vi "FA_Open.vi"(7 "LSCollections":T1, 8 "Error In":errorcluster, 10 "Special Types Array":T2[](array[typedef])) -> (0 "Error Out":errorcluster, 3 "FA_LS Ref":T3)   [LabVIEW 2014, in "FA_LocalStore.lvlib"]
doc: "Opens a reference to the XML files for each Special Type configuraiton. Implicitely opens reference to FA_eTag."
uses:
  FA_LocalStore.lvlib
  FA_LSRef.ctl
  <vilib>/Utility/config.llb/Config Data RefNum.ctl
  FA_LSSpecialTypes.ctl
  FA_LSCollections.ctl
  <vilib>/Utility/config.llb/NI_LVConfig.lvlib
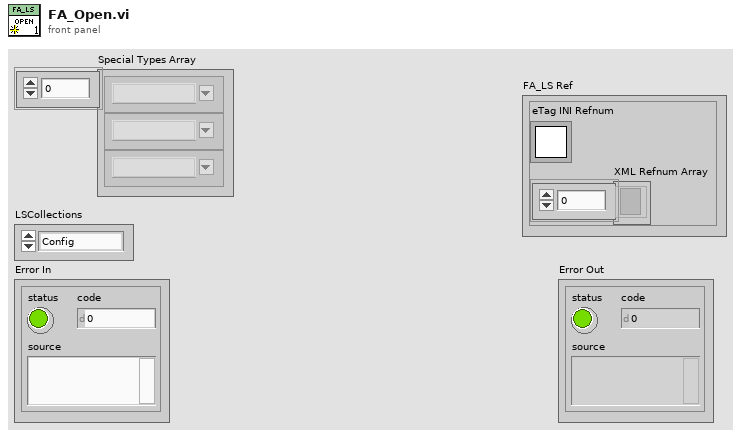
[diagram p1: front panel]
types:
  T1 = typedef "FA_LocalStore.lvlib/FA_LSCollections.ctl" = enum16{"Config", "ConfigItem", "FA_eTag", "FA_PlugIn"}
  T2 = typedef "FA_LocalStore.lvlib/FA_LSSpecialTypes.ctl" = string
  T3 = typedef "FA_LocalStore.lvlib/FA_LSRef.ctl" = cluster{"eTag INI Refnum":T4, "XML Refnum Array":refnum<file>[]}
  T4 = typedef "NI_LVConfig.lvlib/Config Data RefNum.ctl" = refnum<k1>
  T5 = enum16{"open", "replace", "create", "open or create", "replace or create", "replace or create with confirmation"}
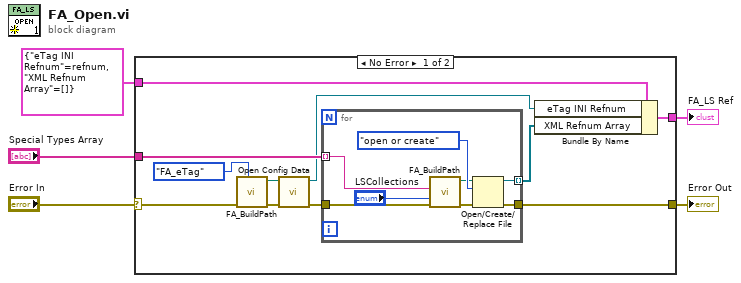
[diagram p0: block diagram]
diagram:
  n1 = case shown="No Error" "Error In" {
    selector: "Error In" -> [w14 w25]
    tunnel: [w16 w25] -> w4
    tunnel: "Special Types Array" -> [w15 _]
    tunnel: T3 {"eTag INI Refnum"=refnum, "XML Refnum Array"=[]} ("FA_LS Ref") -> [w9 _]
    tunnel: [w6 _] -> w1
    frame No Error {
      n2 = call "FA_BuildPath.vi"("LSCollections"=FA_LSCollections."FA_eTag", "error in (no error)"=w14) -> ("error out"=w13:errorcluster, "file path"=w11:path)  [unwired: 7 in, 1 out]
      n3 = call <vilib>:"Open Config Data.vi"("error in (no error)"=w13, "configuration file path"=w11) -> ("error out"=w12:errorcluster, "refnum"=w7:T4)  [unwired: 7 in, 1 out]
      n4 = for {
        tunnel: w12 -> [w23]
        tunnel: [w24] -> w16
        tunnel: w15 -> [w20] mode=indexing
        tunnel: [w17] -> w8 mode=indexing
        n5 = call "FA_BuildPath.vi"("LSCollections"="LSCollections", "error in (no error)"=w23, "Special Type"=w20) -> ("error out"=w22:errorcluster, "file path"=w19:path)  [unwired: 6 in, 1 out]
        n6 = Open/Create/Replace File(file path (use dialog)=w19, error in=w22, operation (0:open)=T5."open or create") -> (refnum out=w17:refnum<file>, error out=w24:errorcluster)  [unwired: 3 in, 1 out]
      }
      n7 = Bundle By Name(cluster=w9, "eTag INI Refnum"=w7, "XML Refnum Array"=w8) -> (w6:T3)
    }
    frame Error {
    }
  }
  "FA_LS Ref" <- w1
  "Error Out" <- w4
